vi "Move DC_2_Power.vi"(2 "DC Motors":T2={"DC Motor"=enum."DC Motor", "Address"=-1, "Address"=-1}, 3 "NXT":T3={"Hardware"="NXT", "Flattened String"=""}, 4 "Power1 (100)":i8=100, 8 "Power2 (100)":i8=100) -> (0 "NXT":T3={"Hardware"="NXT", "Flattened String"=""})   [LabVIEW 2010, in "4134Outputs.lvlib"]
uses:
  4134Outputs.lvlib
  <vilib>/NXT/Subs/LVHSConnector.ctl
  <vilib>/NXT/Subs/MotorXNode.DC Motor Type.ctl
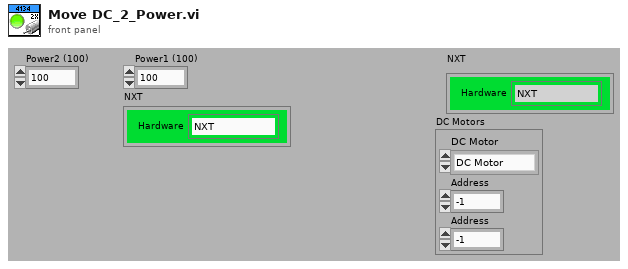
[diagram p1: front panel]
types:
  T1 = typedef "MotorXNode.DC Motor Type.ctl" = enum16{"DC Motor"}
  T2 = cluster{"DC Motor":T1, "Address":i16, "Address":i16}
  T3 = typedef "LVHSConnector.ctl" = cluster{"Hardware":string, "Flattened String":string}
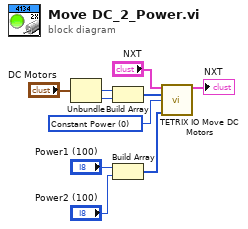
[diagram p0: block diagram]
diagram:
  w6 = u8 0 items=["Constant Power", "Constant Speed"] ("Control Mode (Constant Power)")
  n1 = Unbundle("DC Motors") -> ("Address"=w10:i16, "Address"=w2:i16)  [unwired: 1 out]
  n2 = Build Array(w10, w2) -> (w9:i16[])
  n3 = Build Array("Power1 (100)", "Power2 (100)") -> (w7:i8[])
  n4 = call <vilib>:"TETRIX IO Move DC Motors.vi"("NXT"="NXT", "DC Motors"=w9, "Control Mode (Constant Power)"=w6, "Power / Speed"=w7) -> ("NXT"=→"NXT":T3)  [unwired: 11 in]
